vi "AddHeaderCheckSumAndConvert.vi"(11 "unsigned byte array":u8[](array[numeric])=[170, 85]) -> (1 "string":string, 2 "string 2":string, 3 "size(s) 3":u8)   [LabVIEW 2018]
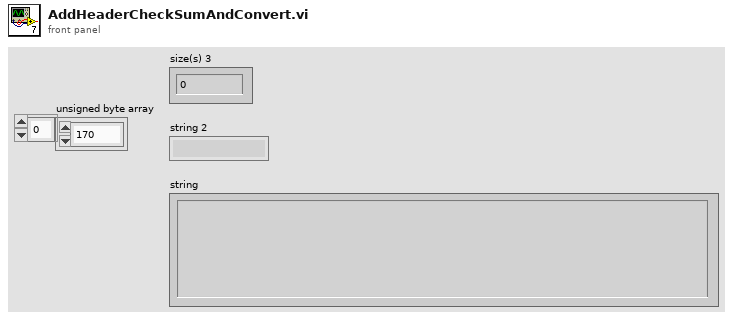
[diagram p1: front panel]
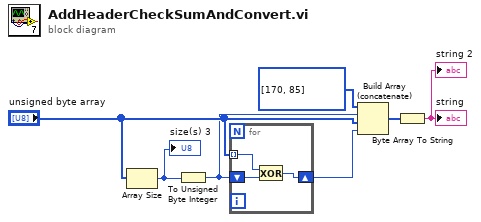
[diagram p0: block diagram]
diagram:
  n1 = Array Size(array="unsigned byte array") -> (size(s)=w5:i32)
  "size(s) 3" <- w5
  n2 = To Unsigned Byte Integer(number=w5) -> (unsigned 8bit integer=w2:u8)
  n3 = for {
    tunnel: "unsigned byte array" -> [w10] mode=indexing
    shift-right: [w9] -> w1
    shift-left: w2 -> [w8]
    n4 = Exclusive Or(1:w8, 2:w10) -> (0:w9:u8)
  }
  n5 = Build Array (concatenate)(u8[] [170, 85] ("unsigned byte array"), w2, "unsigned byte array", w1) -> (w6:u8[])
  n6 = Byte Array To String(unsigned byte array=w6) -> (string=→"string" →"string 2":string)
